vi "AsynchronousScriptHelper.vi"   [LabVIEW 2011]
uses:
  <vilib>/Rock Robotics/WPI/DriverStation/WPI_DriverStationStatusErrorCache.ctl
  MutexMode.ctl
panel:
  # "Helper reads the calling script name from the datastore and executes the script\nThe purpose of this is to allow calling of a static VI ref with no front panel objects"
types:
  T1 = typedef "WPI_DriverStationStatusErrorCache.ctl" = enum16{"Get", "Set"}
  T2 = typedef "MutexMode.ctl" = enum16{"Get Mode", "Request Execution", "Stop Execution", "Lock Autonomous", "Script Completed"}
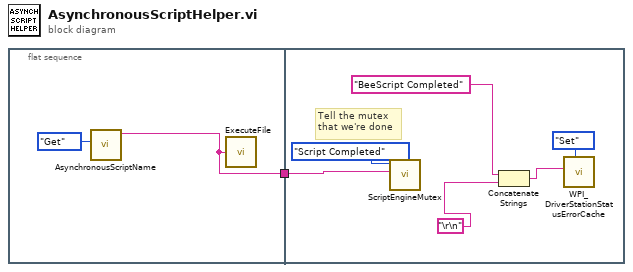
[diagram p0: block diagram]
diagram:
  n1 = flat-sequence {
    tunnel: [w2] -> w1
    tunnel: w1 -> [w8]
    frame #0 {
      n2 = call "AsynchronousScriptName.vi"("data_store_mode"=enum16{"Set", "Get"}."Get") -> ("Call Script"=w2:string)  [unwired: 10 in]
      n3 = call "ExecuteFile.vi"("File Name With Extension"=w2) -> ()
    }
    frame #1 {
      # "Tell the mutex\nthat we're done"
      n4 = call "ScriptEngineMutex.vi"("Calling Script"=w8, "Mutex Mode"=MutexMode."Script Completed") -> ()  [unwired: 9 in, 1 out]
      n5 = Concatenate Strings("BeeScript Completed" ("string"), "\r\n") -> (w7:string)
      n6 = call <vilib>:"WPI_DriverStationStatusErrorCache.vi"("StatusErrorCacheOp"=WPI_DriverStationStatusErrorCache."Set", "Error String"=w7) -> ()  [unwired: 10 out]
    }
  }
